vi "Read Person.vi"(11 "People Wrapper in":refnum<class "People By Year Wrapper.lvclass">) -> (2 "Person":T1 {"Birth Date" format="%<%Y/%b/%d>T"})   [LabVIEW 2023, in "People By Year Wrapper.lvclass"]
uses:
  People By Year Wrapper.lvclass
  Person Information.ctl
  People By Year Wrapper.lvclass/People By Year Wrapper.ctl
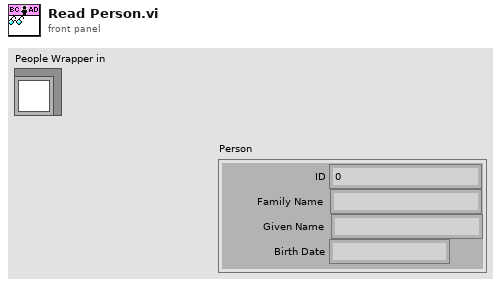
[diagram p1: front panel]
types:
  T1 = typedef "Person Information.ctl" = cluster{"ID":u32, "Family Name":string, "Given Name":string, "Birth Date":timestamp}
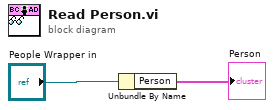
[diagram p0: block diagram]
diagram:
  n1 = Unbundle By Name("People Wrapper in") -> ("Person"=→"Person":T1)
